vi "Flood Glyph.vi"(6 "Use New Fill Algorithm? (F)":bool, 11 "image data":T1) -> (3 "Pic Out":picture)   [LabVIEW 2020, in "lv_icon.lvlib"]
doc: "This VI is used to get rid of transparency within a shape where it actually should be filled with white."
uses:
  resource/plugins/lv_icon.lvlib
  <vilib>/picture/picture.llb/imagedata.ctl
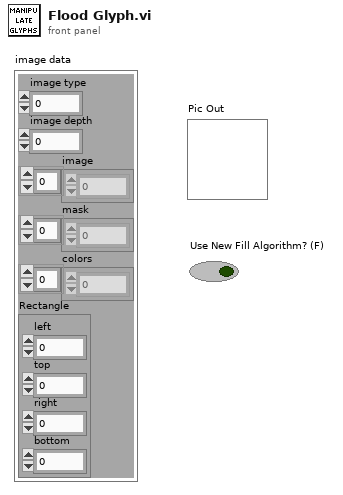
[diagram p1: front panel]
types:
  T1 = typedef "imagedata.ctl" = cluster{"image type":i32, "image depth":i32, "image":u8[], "mask":u8[], "colors":u32[], "Rectangle":cluster{"left":i16, "top":i16, "right":i16, "bottom":i16}}
  T2 = cluster{"left":i16, "top":i16, "right":i16, "bottom":i16}
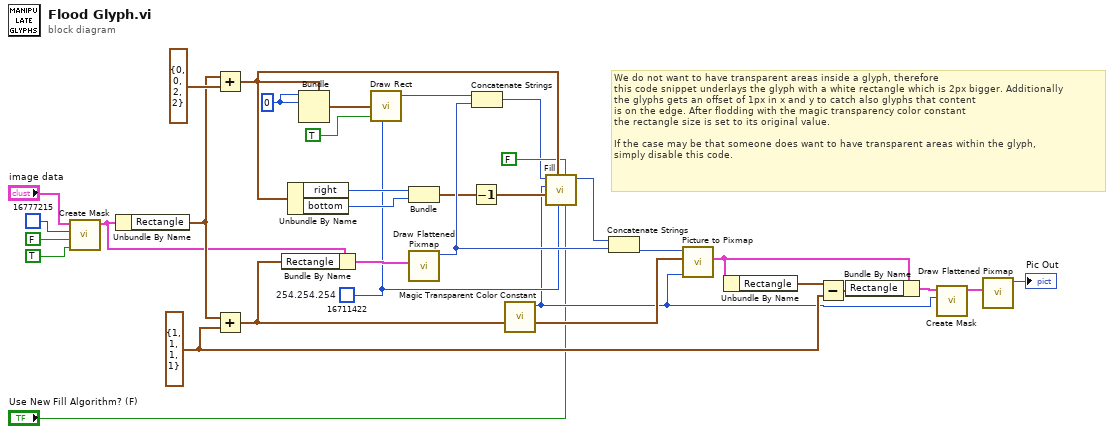
[diagram p0: block diagram]
diagram:
  w23 = i16 0 ("left")
  w21 = u32 16711422  # 254.254.254
  w12 = T2 {"left"=1, "top"=1, "right"=1, "bottom"=1} ("y")
  # "We do not want to have transparent areas inside a glyph, therefore\nthis code snippet underlays the glyph with a white rectangle which is 2px bigger. Additionally\nthe glyphs gets an offset of 1px in x and y to catch also glyphs that content\nis on the edge. After flodding with the magic transparency color constant\nthe rectangle size is set to its original value.\n\nIf the case may be that someone does want to have transparent areas within the glyph,\nsimply disable this code."
  n1 = call <vilib>:"Create Mask.vi"("Combine Masks? (F)"=TRUE, "1-Bit Mask Value (T)"=FALSE, "Mask Color (Black)"=u32 16777215, "image data"="image data") -> ("image data"=w7:T1)  [unwired: 7 out]
  n2 = Unbundle By Name(w7) -> ("Rectangle"=w18:T2)
  n3 = Add(x=w18, y=T2 {"left"=0, "top"=0, "right"=2, "bottom"=2}) -> (x+y=w24:T2)
  n4 = Add(x=w18, y=w12) -> (x+y=w19:T2)
  n5 = Bundle By Name(cluster=w7, "Rectangle"=w19) -> (w28:T1)
  n6 = Unbundle By Name(w24) -> ("right"=w30:i16, "bottom"=w31:i16)
  n7 = Bundle(cluster=w24, "left"=w23, "top"=w23) -> (w22:T2)  [unwired: 2 out]
  n8 = call <vilib>:"Draw Rect.vi"("rect"=w22, "fill?(F)"=TRUE, "color(black)"=w21) -> ("new picture"=w32:picture)  [unwired: 2 in, 4 out]
  n9 = Bundle("right"=w30, "bottom"=w31) -> (w20:cluster{"right":i16, "bottom":i16})  [unwired: 1 out]
  n10 = call <vilib>:"Draw Flattened Pixmap.vi"("image data"=w28) -> ("new picture"=w27:picture)  [unwired: 1 in, 7 out]
  n11 = Decrement(x=w20) -> (x-1=w17:cluster{"right":i16, "bottom":i16})
  n12 = Concatenate Strings(w32, w27) -> (w5:picture)
  n13 = call "Magic Transparent Color Constant.vi"() -> ("Magic transparent color constant"=w8:u32)  [unwired: 11 out]
  n14 = call "Fill.vi"("Use New Fill Algorithm? (F)"="Use New Fill Algorithm? (F)", "Tool filling? (T)"=FALSE, "Ref Color"=w21, "rect"=w24, "Pic Mouse Down"=w17, "New Color"=w8, "Pic In"=w5) -> ("Pic Out"=w16:picture)  [unwired: 4 out]
  n15 = Concatenate Strings(w16, w27) -> (w25:picture)
  n16 = call <vilib>:"Picture to Pixmap.vi"("Background Color"=w8, "rect"=w19, "picture"=w25) -> ("image data"=w11:T1)  [unwired: 1 in, 7 out]
  n17 = Unbundle By Name(w11) -> ("Rectangle"=w13:T2)
  n18 = Subtract(x=w13, y=w12) -> (x-y=w10:T2)
  n19 = Bundle By Name(cluster=w11, "Rectangle"=w10) -> (w9:T1)
  n20 = call <vilib>:"Create Mask.vi"("Mask Color (Black)"=w8, "image data"=w9) -> ("image data"=w15:T1)  [unwired: 2 in, 7 out]
  n21 = call <vilib>:"Draw Flattened Pixmap.vi"("image data"=w15) -> ("new picture"=→"Pic Out":picture)  [unwired: 1 in, 7 out]
